vi "SAC-Configure Hardware (NI).vi"(0 "Params":T1={"Fs (Hz)"=0.0, "atten (dB)"=0.0, "Waveform"=enum."Chirp", "Freq Res (Hz)"=0.0, "Order"=0, "Averages"=0, "seed"=-1, "Window"={"Type"=enum."None", "Length (ms)"=0.0, "Center (ms)"=0.0}, "Mic gain"=0.0, "Mic sens"=0.0}, 11 "error in (no error)":errorcluster) -> (4 "Stimulus":dbl[](array[numeric]), 6 "Sample Rate (Hz)":dbl, 8 "pts/rep":i32, 10 "reps/frame":i32, 15 "error out":errorcluster)   [LabVIEW 2020]
uses:
  Typedefs/SAC-Parameters.ctl
  HRTF VIs/Typedefs/HRTF-Waveform.ctl
  HRTF VIs/Typedefs/HRTF-Window.ctl
  HRTF VIs/Typedefs/HRTF-Window Type.ctl
  Utility VIs/Math VIs/dB to Linear (scalar).vi
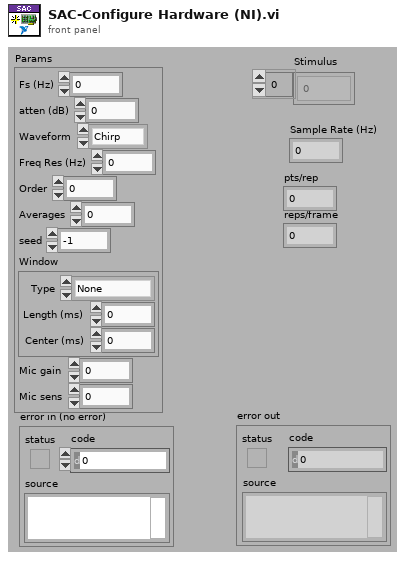
[diagram p1: front panel]
types:
  T1 = typedef "SAC-Parameters.ctl" = cluster{"Fs (Hz)":dbl, "atten (dB)":dbl, "Waveform":T2, "Freq Res (Hz)":dbl, "Order":i32, "Averages":i32, "seed":i64, "Window":T3, "Mic gain":dbl, "Mic sens":dbl}
  T2 = typedef "HRTF-Waveform.ctl" = enum16{"Chirp", "MLS"}
  T3 = typedef "HRTF-Window.ctl" = cluster{"Type":T4, "Length (ms)":dbl, "Center (ms)":dbl}
  T4 = typedef "HRTF-Window Type.ctl" = enum16{"None", "Rectangle", "Hanning"}
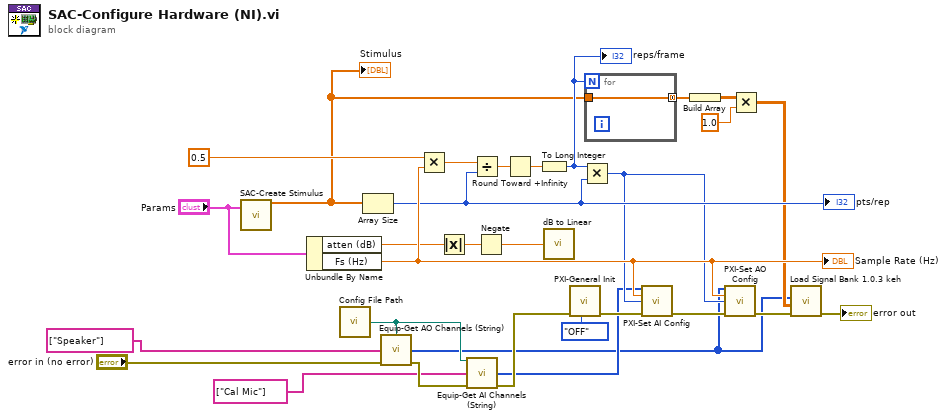
[diagram p0: block diagram]
diagram:
  n1 = call "SAC-Create Stimulus.vi"("Params"="Params") -> ("Stimulus"=w10:dbl[])  [unwired: 9 in, 5 out]
  "Stimulus" <- w10
  n2 = Unbundle By Name("Params") -> ("atten (dB)"=w13:dbl, "Fs (Hz)"=w22:dbl)
  "Sample Rate (Hz)" <- w22
  n3 = call "Config File Path.vi"() -> ("Default config file name"=w7:path)  [unwired: 1 in]
  n4 = Array Size(array=w10) -> (size(s)=w20:i32)
  "pts/rep" <- w20
  n5 = call "Equip-Get AO Channels (String).vi"("Path"=w7, "Channel Names"=string[] ["Speaker"] ("Requested Endpoints"), "error in (no error)"="error in (no error)") -> ("AO Channels"=w3:i32[], "error out"=w6:errorcluster)  [unwired: 11 in]
  n6 = Multiply(x=0.5, y=w22) -> (x*y=w21:dbl)
  n7 = Absolute Value(x=w13) -> (abs(x)=w12:dbl)
  n8 = call "Equip-Get AI Channels (String).vi"("Path"=w7, "Inputs"=string[] ["Cal Mic"] ("Requested Endpoints"), "error in (no error)"=w6) -> ("AI Channels"=w4:i32[], "error out"=w5:errorcluster)  [unwired: 11 in]
  n9 = Divide(x=w21, y=w20) -> (x/y=w24:dbl)
  n10 = Negate(x=w12) -> (-x=w11:dbl)
  n11 = Round Toward +Infinity(x=w24) -> (ceil(x): smallest int >= x=w23:dbl)
  n12 = To Long Integer(number=w23) -> (32bit integer=w17:i32)
  "reps/frame" <- w17
  n13 = call-poly "dB to Linear.vi"("dB"=w11) -> ()  [unwired: 1 out]
  n14 = call "PXI-General Init.vi"("Double Buffer Mode"=enum32{"OFF", "ENABLED", "FORCED"}."OFF", "error in (no error)"=w5) -> ("error out"=w29:errorcluster)  [unwired: 9 in]
  n15 = Multiply(x=w17, y=w20) -> (x*y=w19:i32)
  n16 = for {
    N: w17 -> [_]
    tunnel: w10 -> [w31]
    tunnel: [w31] -> w16 mode=concatenating
  }
  n17 = call "PXI-Set AI Config.vi"("AI Channels"=w4, "Sampling Rate (Hz)"=w22, "Buffer Size"=w19, "error in (no error)"=w29) -> ("error out"=w28:errorcluster)  [unwired: 11 in]
  n18 = Build Array(w16) -> (w26:dbl[][])
  n19 = call "PXI-Set AO Config.vi"("AO Channels"=w3, "Sampling Rate (Hz)"=w22, "Buffer Size"=w19, "error in (no error)"=w28) -> ("error out"=w27:errorcluster)  [unwired: 11 in]
  n20 = Multiply(x=w26, y=1.0) -> (x*y=w14:dbl[][])
  n21 = call "Load Signal Bank 1.0.3 keh.vi"("error in (no error)"=w27, "Input array"=w14, "Active AO Array"=w3) -> ("error out"=→"error out":errorcluster)  [unwired: 6 in, 2 out]
